vi "set_multipart_form.vi"(8 "error in (no error)":errorcluster, 10 "MultipartForm":refnum<class "MultipartForm.lvclass">, 11 "RequestBuilder in":refnum<class "RequestBuilder.lvclass">) -> (0 "error out":errorcluster, 2 "success":bool, 3 "RequestBuilder out":refnum<class "RequestBuilder.lvclass">)   [LabVIEW 2020, in "reqwest.lvlib" / "RequestBuilder.lvclass"]
uses:
  RequestBuilder.lvclass
  RequestBuilder.lvclass/RequestBuilder.ctl
  MultipartForm/MultipartForm.lvclass
  lv_reqwest_64.dll
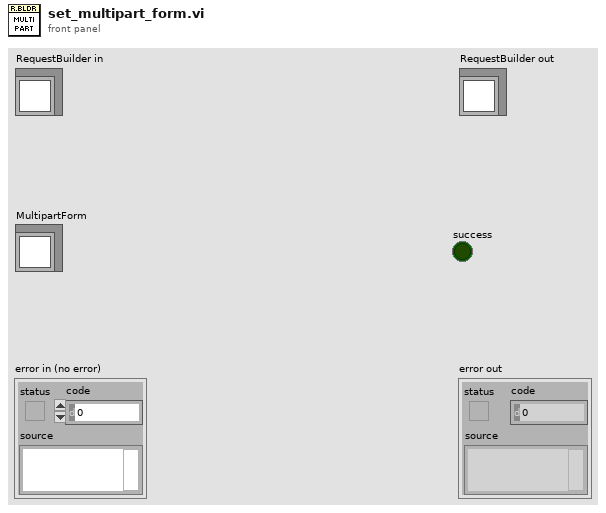
[diagram p1: front panel]
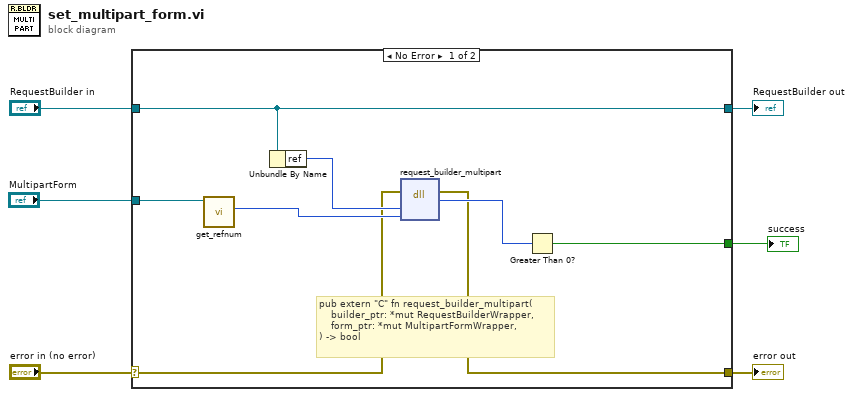
[diagram p0: block diagram]
diagram:
  n1 = case shown="No Error" "error in (no error)" {
    selector: "error in (no error)" -> [w8 w16]
    tunnel: [w7 w16] -> w5
    tunnel: [w11 w15] -> w3
    tunnel: "RequestBuilder in" -> [w11 w15]
    tunnel: "MultipartForm" -> [w14 _]
    tunnel: [w9 _] -> w1
    frame No Error {
      # "pub extern \"C\" fn request_builder_multipart(\n    builder_ptr: *mut RequestBuilderWrapper,\n    form_ptr: *mut MultipartFormWrapper,\n) -> bool"
      n2 = call "get_refnum.vi"("MultipartForm"=w14) -> ("ref"=w12:u64)  [unwired: 10 in]
      n3 = Unbundle By Name(w11) -> ("ref"=w10:u64)
      n4 = dll-call lib="C:/Projects/reqwest-rs-labview/lv_src/lv_reqwest_*.*" fn="request_builder_multipart"(error in=w8, "builder_ptr"=w10, "form_ptr"=w12) -> (error out=w7:errorcluster, "Return Value"=w13:u8)  [unwired: 4 in, 1 out]
      n5 = Greater Than 0?(x=w13) -> (x > 0?=w9:bool)
    }
    frame Error {
    }
  }
  "error out" <- w5
  "RequestBuilder out" <- w3
  "success" <- w1
